vi "Init FPGA Control.vi"(0 "FPGA VI Reference In":refnum<k20>, 1 "Window Function":enum16{"None", "Hanning"}(ring)=enum."Hanning", 2 "n":u32=5, 3 "lower limit 1":u32=113, 4 "lower limit 2":u32=738, 5 "error in":errorcluster, 6 "n-bit (2^(nbit) signals for Residual Extraction)":i32=10, 7 "Initial Latency points":u32=260, 9 "first FFT bin":i32=5, 11 "last FFT bin":i32=255) -> (14 "FPGA VI Reference Out":refnum<k20>, 19 "error out":errorcluster)   [LabVIEW 2014]
uses:
  <vilib>/Utility/error.llb/Error Cluster From Error Code.vi
  <vilib>/rvi/errors/niLvFpgaAdjustHostInterfaceError.vi
  <vilib>/rvi/interface/nirviReadWriteControl/nirviReadWriteControl.xnode
  NiFpgaLv.dll
  <vilib>/rvi/interface/Simulation/niFpgaSimulationCallBeginRW.vi
panel:
  # "PARAMETERS"
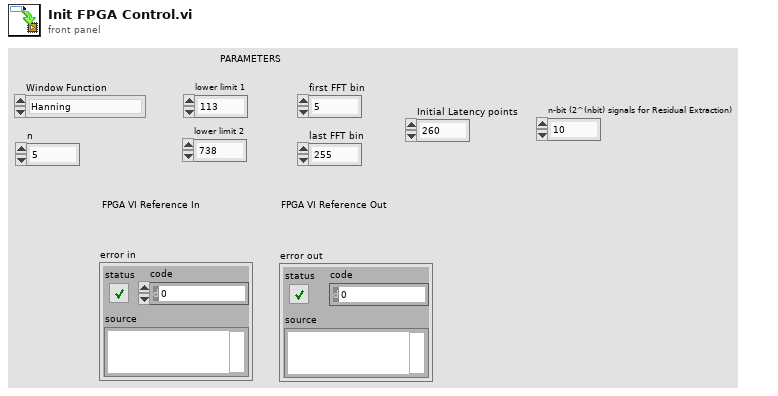
[diagram p1: front panel]
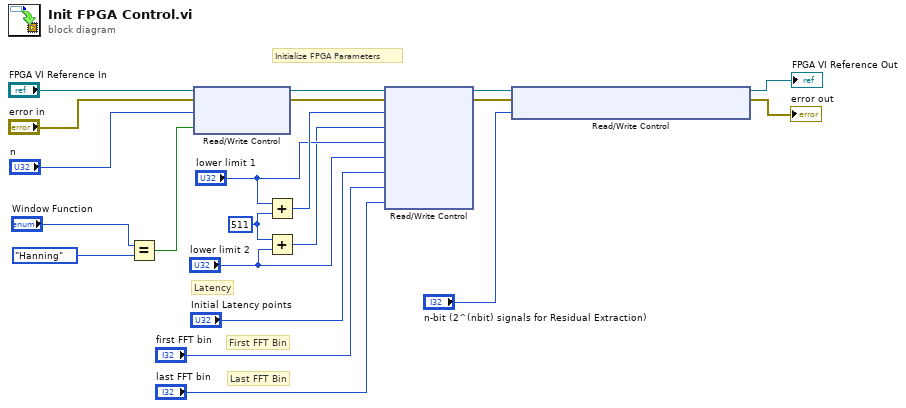
[diagram p0: block diagram]
diagram:
  w11 = u32 511 ("y")
  # "Initialize FPGA Parameters"
  # "Last FFT Bin"
  # "First FFT Bin"
  # "Latency"
  n1 = Equal?(x="Window Function", y=enum16{"None", "Hanning"}."Hanning" ("Windowing")) -> (x = y?=w15:bool)
  n2 = xnode "Read/Write Control"("FPGA VI Reference In"="FPGA VI Reference In", "error in"="error in", "n"="n", "Hanning window"=w15) -> ("FPGA VI Reference Out"=w17:refnum<k20>, "error out"=w16:errorcluster)
  n3 = Add(x="lower limit 1", y=w11) -> (x+y=w21:u32)
  n4 = Add(x=w11, y="lower limit 2") -> (x+y=w19:u32)
  n5 = xnode "Read/Write Control"("FPGA VI Reference In"=w17, "error in"=w16, "upper limit 1"=w21, "upper limit 2"=w19, "lower limit 1"="lower limit 1", "lower limit 2"="lower limit 2", "Latency points"="Initial Latency points", "First bin"="first FFT bin", "Last bin"="last FFT bin") -> ("FPGA VI Reference Out"=w5:refnum<k20>, "error out"=w4:errorcluster)
  n6 = xnode "Read/Write Control"("FPGA VI Reference In"=w5, "error in"=w4, "n-bit (2^(nbit) signals for Residual Extraction)"="n-bit (2^(nbit) signals for Residual Extraction)") -> ("FPGA VI Reference Out"=→"FPGA VI Reference Out":refnum<k20>, "error out"=→"error out":errorcluster)
